vi "DMA T-H FIFO Write U32.vi"(0 "Data In":u32, 1 "FIFO In":refnum<k21>="RX", 5 "Input Valid":bool) -> (4 "Ready for Input?":bool)   [LabVIEW 2012]
doc: "FIFO Write\n\nThis VI is intended to be used as a wrapper around FIFOs. 4 Wire handshaking has been added."
uses:
  <vilib>/rvi/DataTransferAndStorage/Container/Common/niFpgaContainerExecOnDevCompGetState.vi
  <vilib>/rvi/Emulation/niFpgaSctlEmulationGetInTimedLoop.vi
  <vilib>/rvi/DataTransferAndStorage/Container/Common/niFpgaContainerGetUniqueNameForEmu.vi
  <vilib>/rvi/FIFO/Fifo_Resource/nirvififoEmulationSetSize.vi
  <vilib>/rvi/errors/niFpgaSetErrorForExecOnDevCompSimple.vi
  <vilib>/rvi/eio/common/nirviEmuReportErrorAndStop.vi
  <vilib>/rvi/Emulation/niFpgaSctlEmulationFifoFullMgr.vi
  <vilib>/rvi/Emulation/niFpgaSctlEmulationResourceMgr.vi
  <vilib>/rvi/interface/RandomDataEmulation/nirviRandomDataFPGAFIFO.vi
  <vilib>/rvi/interface/RandomDataEmulation/niFpgaRandomDataHandleErrors.vi
  <vilib>/rvi/DataTransferAndStorage/Container/XNode/niFpgaContainer.xnode
  <vilib>/rvi/FIFO/Fifo_Resource/niFpgaFifoEmulationRefIn.vi
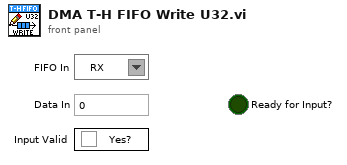
[diagram p1: front panel]
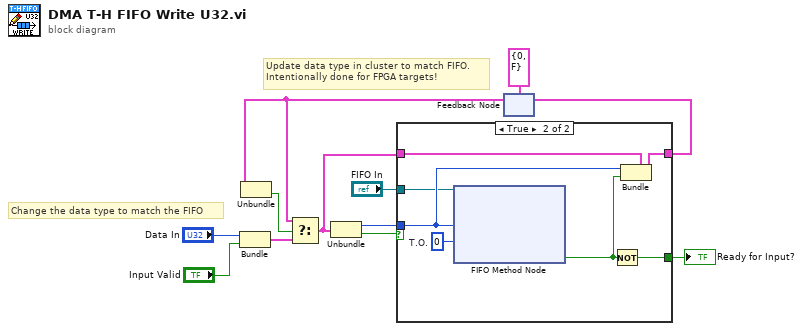
[diagram p0: block diagram]
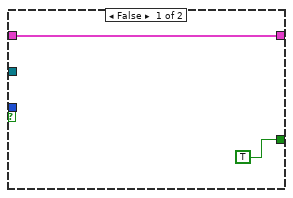
[diagram p2: hidden frame]
diagram:
  # "Update data type in cluster to match FIFO.\nIntentionally done for FPGA targets!"
  # "Change the data type to match the FIFO"
  n1 = Bundle("Data In"="Data In", "Input Valid"="Input Valid") -> (w9:cluster{"Data In":u32, "Input Valid":bool})  [unwired: 1 in]
  n2 = feedback #1(cluster{"Data In":u32, "Input Valid":bool} {"Data In"=0, "Input Valid"=FALSE} ("cluster")) -> (w2:cluster{"Data In":u32, "Input Valid":bool})
  n3 = Unbundle(w2) -> ("Input Valid"=w5:bool)  [unwired: 1 out]
  n4 = Select(t=w2, s=w5, f=w9) -> (s? t:f=w4:cluster{"Data In":u32, "Input Valid":bool})
  n5 = Unbundle(w4) -> ("Data In"=w7:u32, "Input Valid"=w8:bool)
  n6 = case shown="True" w8 {
    tunnel: [TRUE w19] -> w12
    tunnel: w7 -> [_ w17]
    tunnel: w4 -> [w13 w21]
    tunnel: [w13 w20] -> w3
    tunnel: "FIFO In" -> [_ w15]
    frame False {
    }
    frame True {
      w18 = 0  # T.O.
      n7 = xnode ("FIFO Method Node")("Element"=w17, "Timeout"=w18, "FIFO In"=w15) -> ("Timed Out?"=w16:bool)  [unwired: 1 out]
      n8 = Not(x=w16) -> (.not. x?=w19:bool)
      n9 = Bundle(cluster=w21, "Data In"=w17, "Input Valid"=w16) -> (w20:cluster{"Data In":u32, "Input Valid":bool})
    }
  }
  "Ready for Input?" <- w12
  n10 = feedback-in #1(w3) -> ()
